vi "Is Latched Boolean.vi"(8 "error in":errorcluster, 11 "control in":refnum<vi>) -> (0 "error out":errorcluster, 2 "is latched boolean":bool, 3 "control out":refnum<vi>)   [LabVIEW 2021, in "NI Measurement Plug-In SDK.lvlib"]
uses:
  NI Measurement Plug-In SDK.lvlib
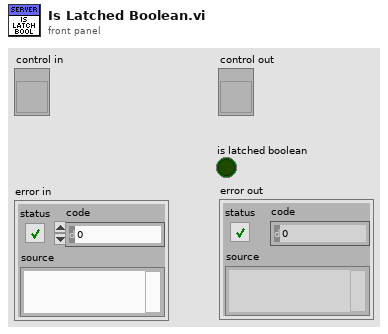
[diagram p1: front panel]
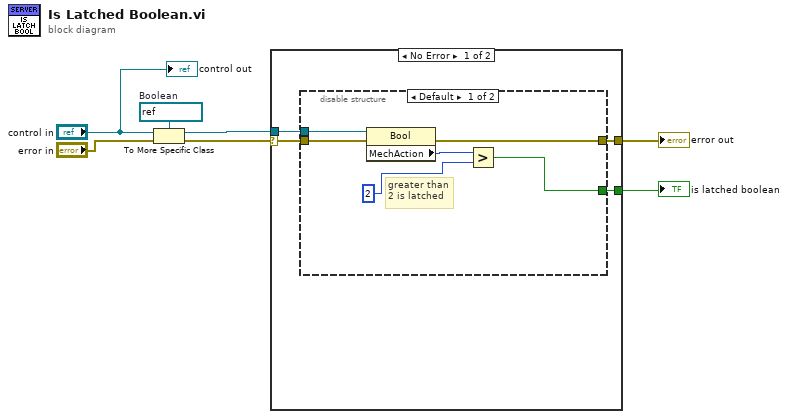
[diagram p0: block diagram]
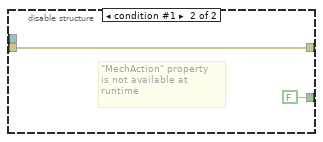
[diagram p2: hidden frame]
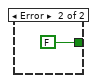
[diagram p3: hidden frame]
diagram:
  w7 = refnum<vi> refnum  # Boolean
  n1 = To More Specific Class(target class=w7, reference="control in", error in="error in") -> (specific class reference=w5:refnum<vi>, error out=w6:errorcluster)
  n2 = case shown="No Error" w6 {
    selector: w6 -> [w9 _]
    tunnel: w5 -> [w10 _]
    tunnel: [w11 FALSE] -> w4
    tunnel: [w8 _] -> w3
    frame No Error {
      n3 = disable-structure shown="Default" {
        disable-tunnel: [w12 FALSE] -> w11
        disable-tunnel: w10 -> [w15 _]
        disable-tunnel: w9 -> [w14 w18]
        disable-tunnel: [w13 w18] -> w8
        frame condition #0 (active) {
          # "greater than\n2 is latched"
          n4 = property class="Bool"(reference=w15, error in=w14) -> (error out=w13:errorcluster, "MechAction"=w17:u32)  [unwired: 1 out]
          n5 = Greater?(x=w17, y=u32 2) -> (0:w12:bool)
        }
        frame condition #1 {
          # "\"MechAction\" property\nis not available at\nruntime"
        }
      }
    }
    frame Error {
    }
  }
  "error out" <- w3
  "is latched boolean" <- w4
  "control out" <- "control in"
